vi "Save VI Info.vi"(8 "error in (no error)":errorcluster, 10 "path":path, 11 "node ref":refnum<vi>) -> (0 "error out":errorcluster, 2 "path out":path, 3 "reference out":refnum<vi>)   [LabVIEW 2014, in "lvprj2html.lvlib"]
uses:
  lvprj2html.lvlib
panel:
  in  "VI Type":T1(ring)
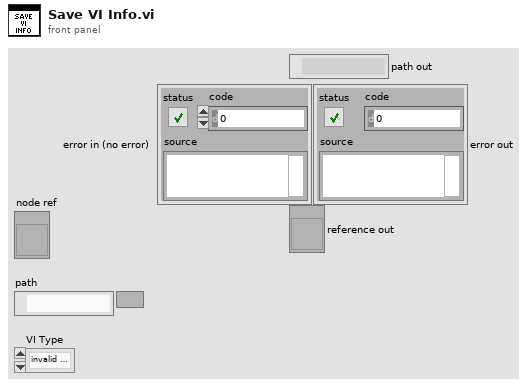
[diagram p1: front panel]
types:
  T1 = enum32{"invalid VI type", "Standard VI", "Control VI", "Global VI", "Polymorphic VI", "Configuration VI", "SubSystem", "Facade VI", "Method VI", "Statechart Diagram VI"}
  T2 = enum16{"open", "replace", "create", "open or create", "replace or create", "replace or create with confirmation"}
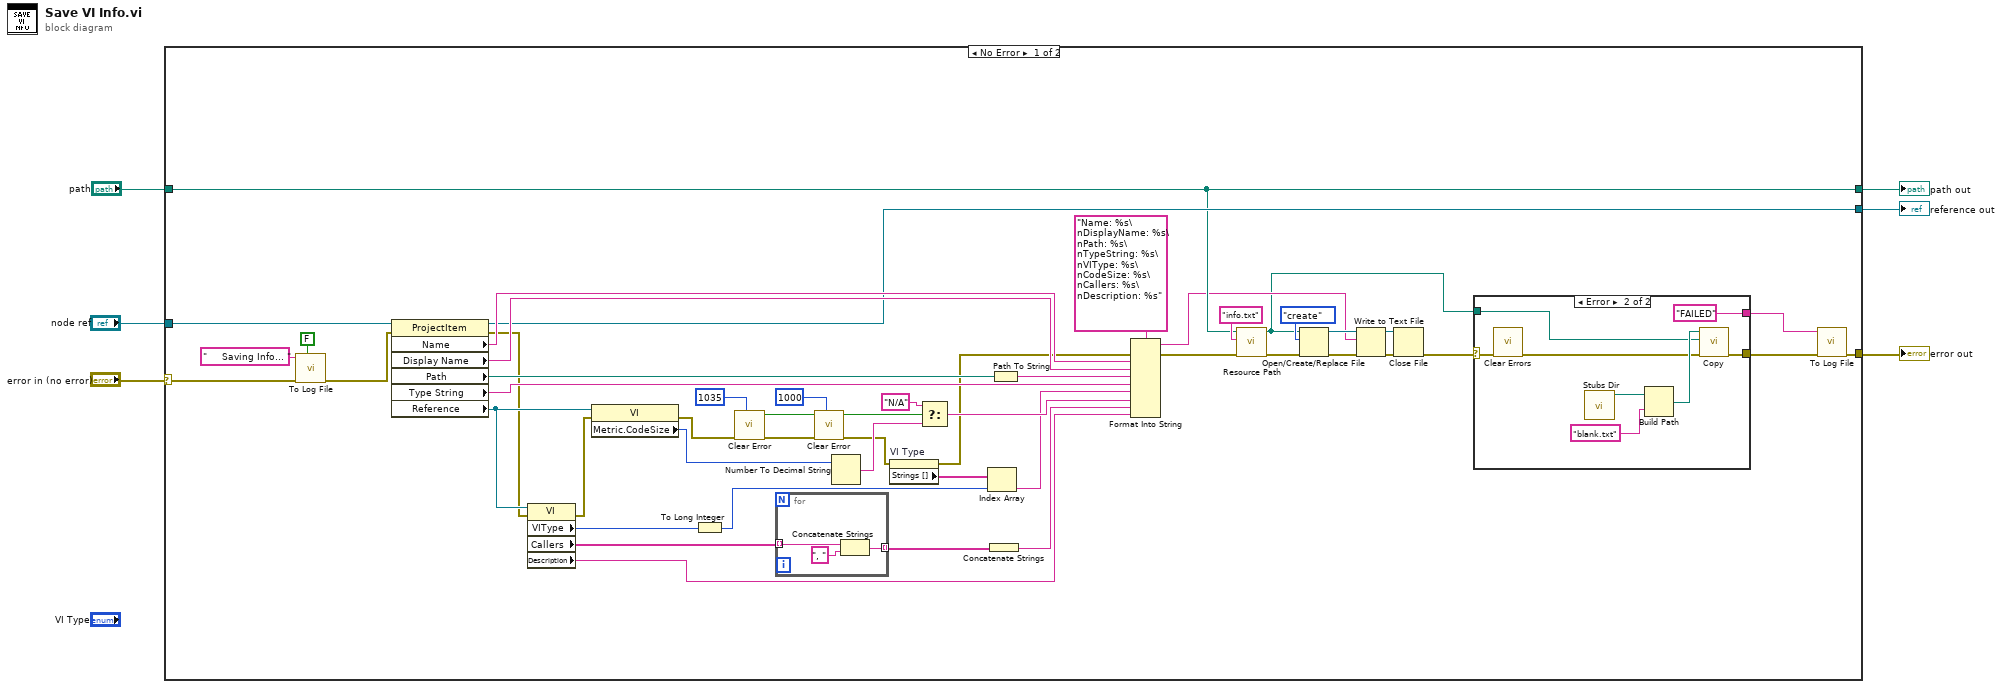
[diagram p0: block diagram]
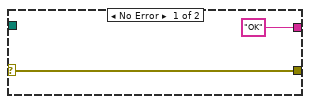
[diagram p2: hidden frame]
diagram:
  n1 = case shown="No Error" "error in (no error)" {
    selector: "error in (no error)" -> [w18 w72]
    tunnel: "node ref" -> [w56 w71]
    tunnel: "path" -> [w17 w70]
    tunnel: [w22 w71] -> w4
    tunnel: [w8 w72] -> w3
    tunnel: [w17 w70] -> w1
    frame No Error {
      n2 = call "To Log File.vi"("new line"=FALSE, "error in (no error)"=w18, "string"="     Saving Info... " ("format string")) -> ("error out"=w19:errorcluster)  [unwired: 8 in]
      n3 = property class="ProjectItem"(reference=w56, error in=w19) -> (reference out=w22:refnum<vi>, error out=w26:errorcluster, "Name"=w34:string, "Display Name"=w33:string, "Path"=w36:path, "Type String"=w37:string, "Reference"=w55:refnum<vi>)
      n4 = property class="VI"(reference=w55, error in=w26) -> (error out=w25:errorcluster, "VIType"=w42:T1, "Callers"=w40:string[], "Description"=w43:string)  [unwired: 1 out]
      n5 = property class="VI"(reference=w55, error in=w25) -> (error out=w46:errorcluster, "Metric.CodeSize"=w45:u32)  [unwired: 1 out]
      n6 = To Long Integer(number=w42) -> (32bit integer=w39:i32)
      n7 = call "Clear Error.vi"("code"=1035, "error in (no error)"=w46) -> ("error out"=w50:errorcluster, "clear"=w53:bool)  [unwired: 8 in]
      n8 = for {
        tunnel: w40 -> [w69] mode=indexing
        tunnel: [w67] -> w41 mode=indexing
        n9 = Concatenate Strings(w69, ", ") -> (w67:string)
      }
      n10 = call "Clear Error.vi"("code"=1000, "error in (no error)"=w50, "prev clear"=w53) -> ("error out"=w24:errorcluster, "clear"=w54:bool)  [unwired: 7 in]
      n11 = Number To Decimal String(number=w45) -> (decimal integer string=w47:string)  [unwired: 1 in]
      n12 = property on="VI Type" class="Enum (strict)"(error in=w24) -> (error out=w16:errorcluster, "Strings []"=w28:string[])  [unwired: 1 in, 1 out]
      n13 = Select(t="N/A", s=w54, f=w47) -> (s? t:f=w49:string)
      n14 = Index Array(array=w28, index=w39) -> (element=w27:string)
      n15 = Concatenate Strings(w41) -> (w44:string)
      n16 = Path To String(path=w36) -> (string=w38:string)
      n17 = Format Into String(format string="Name: %s\nDisplayName: %s\nPath: %s\nTypeString: %s\nVIType: %s\nCodeSize: %s\nCallers: %s\nDescription: %s", error in=w16, w34, w33, w38, w37, w27, w49, w44, w43) -> (resulting string=w12:string, error out=w13:errorcluster)  [unwired: 1 in]
      n18 = call "Resource Path.vi"("error in (no error)"=w13, "resource file name"="info.txt", "data dir"=w17) -> ("error out"=w15:errorcluster, "path"=w7:path)  [unwired: 7 in]
      n19 = Open/Create/Replace File(file path (use dialog)=w7, error in=w15, operation (0:open)=T2."create") -> (refnum out=w30:refnum<file>, error out=w14:errorcluster)  [unwired: 3 in, 1 out]
      n20 = Write to Text File(file (use dialog)=w30, text=w12, error in=w14) -> (refnum out=w31:refnum<file>, error out=w23:errorcluster)  [unwired: 1 in, 1 out]
      n21 = Close File(refnum=w31, error in=w23) -> (error out=w9:errorcluster)  [unwired: 1 out]
      n22 = case shown="Error" w9 {
        selector: w9 -> [w58 w66]
        tunnel: [w58 w60] -> w10
        tunnel: ["OK" ("string") "FAILED" ("string")] -> w11
        tunnel: w7 -> [_ w62]
        frame No Error {
        }
        frame Error {
          n23 = call <vilib>:"Clear Errors.vi"("error in (no error)"=w66) -> ("error out"=w61:errorcluster)  [unwired: 5 in, 1 out]
          n24 = call "Stubs Dir.vi"() -> ("path"=w59:path)  [unwired: 11 in]
          n25 = Build Path(base path=w59, name or relative path="blank.txt") -> (appended path=w63:path)
          n26 = call "Copy.vi"("error in (no error)"=w61, "dst"=w62, "src"=w63) -> ("error out"=w60:errorcluster)  [unwired: 8 in]
        }
      }
      n27 = call "To Log File.vi"("error in (no error)"=w10, "string"=w11) -> ("error out"=w8:errorcluster)  [unwired: 9 in]
    }
    frame Error {
    }
  }
  "error out" <- w3
  "path out" <- w1
  "reference out" <- w4
